vi "Home Stage.vi"(8 "error in (no error)":errorcluster, 11 "2-Axis Stage in":refnum<class "Sync 2-Axis Stage Controller.lvclass">) -> (0 "error out":errorcluster, 3 "2-Axis Stage out":refnum<class "Sync 2-Axis Stage Controller.lvclass">)   [LabVIEW 2022 SP3, in "Sync 2-Axis Stage Controller.lvclass"]
uses:
  Sync 2-Axis Stage Controller.lvclass
  Sync 2-Axis Stage Controller.lvclass/Sync 2-Axis Stage Controller.ctl
  Axis Objects/iMotion Controller/iMotion Controller.lvclass
  Home State.ctl
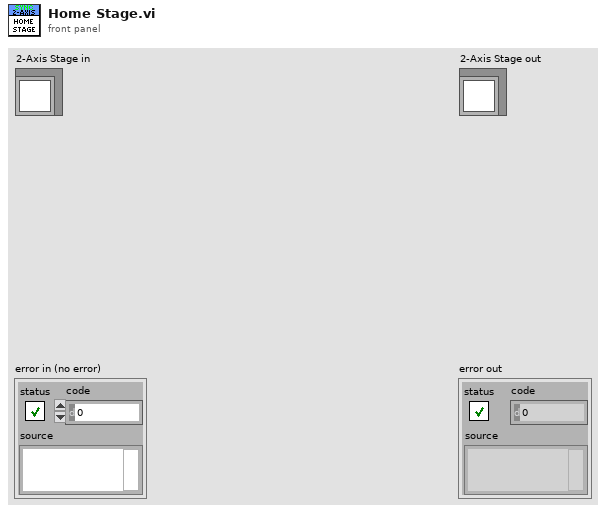
[diagram p1: front panel]
types:
  T1 = typedef "Sync 2-Axis Stage Controller.lvclass/Home State.ctl" = enum16{"Idle", "Homing 1st Axis", "Homing 2nd Axis", "Done"}
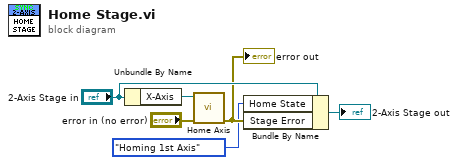
[diagram p0: block diagram]
diagram:
  n1 = Unbundle By Name("2-Axis Stage in") -> ("X-Axis"=w5:refnum<class "iMotion Controller.lvclass">)
  n2 = call-dynamic "Home Axis.vi"("error in (no error)"="error in (no error)", "iMotion Controller in"=w5) -> ("error out"=w3:errorcluster)  [unwired: 8 in, 1 out]
  "error out" <- w3
  n3 = Bundle By Name(cluster="2-Axis Stage in", "Home State"=Home_State."Homing 1st Axis", "Stage Error"=w3) -> (→"2-Axis Stage out":refnum<class "Sync 2-Axis Stage Controller.lvclass">)
